vi "povorot_na_vneshku.vi"() -> ()   [LabVIEW 2017]
uses:
  <vilib>/userdefined/High Color/IMAQdx.ctl
  <vilib>/vision/driver/NI_Vision_Acquisition_Software.lvlib
panel:
  out "X":sgl
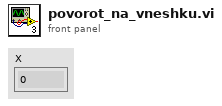
[diagram p1: front panel]
types:
  T1 = typedef "IMAQdx.ctl" = refnum<k21>
  T2 = typedef "IMAQ Image.ctl" = refnum<image>
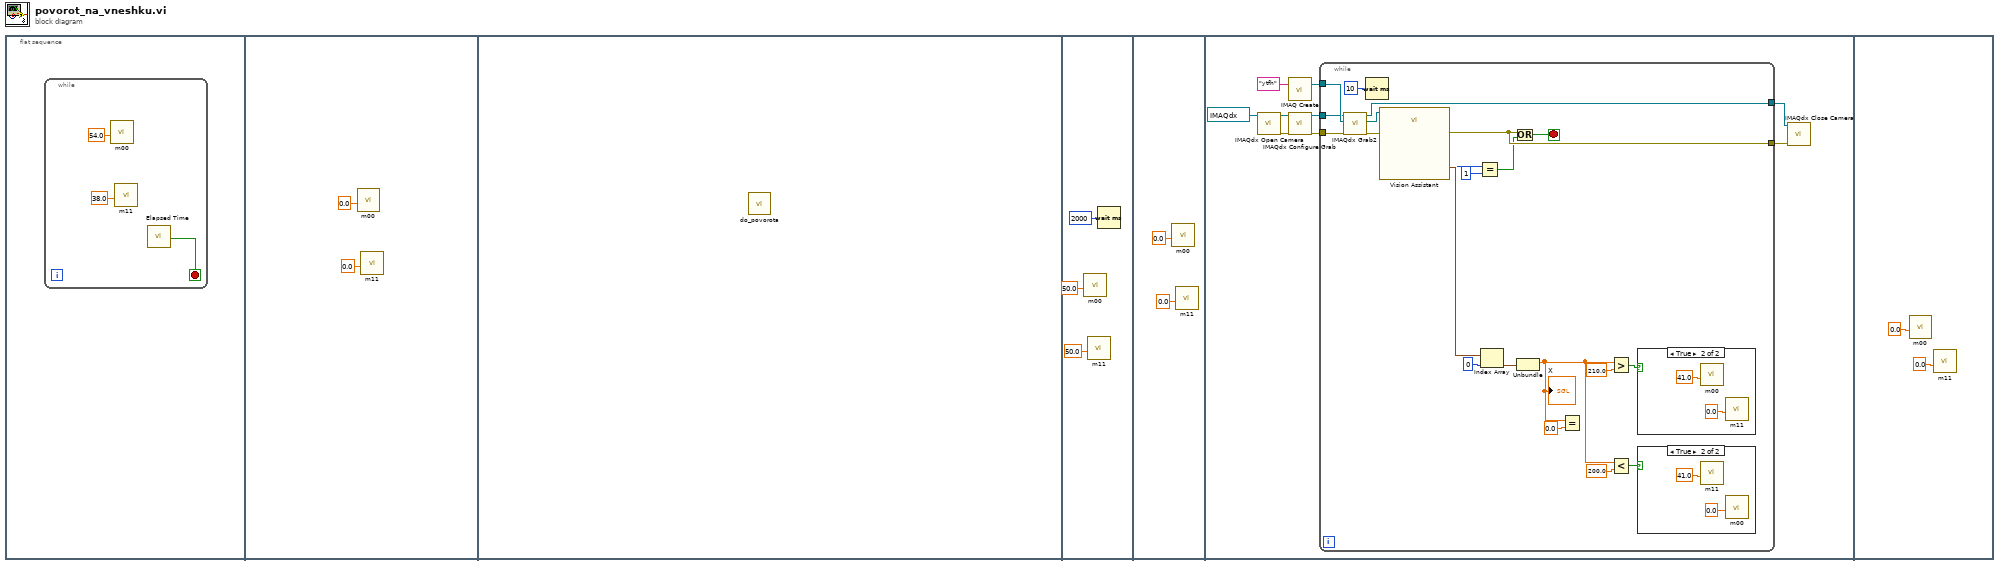
[diagram p0: block diagram]
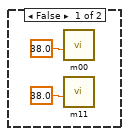
[diagram p2: hidden frame]
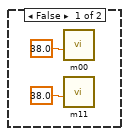
[diagram p3: hidden frame]
diagram:
  n1 = flat-sequence {
    frame #0 {
      n2 = while {
        stop <- w1 stop-if-true
        n3 = call "m00.vi"("position"=54.0) -> ()  [unwired: 10 in, 1 out]
        n4 = call "m11.vi"("position"=38.0) -> ()  [unwired: 10 in, 1 out]
        n5 = call "Elapsed Time"() -> ("Time has Elapsed"=w1:bool)  [unwired: 12 in, 7 out]
      }
    }
    frame #1 {
      n6 = call "m00.vi"("position"=0.0) -> ()  [unwired: 10 in, 1 out]
      n7 = call "m11.vi"("position"=0.0) -> ()  [unwired: 10 in, 1 out]
    }
    frame #2 {
      n8 = call "do_povorota.vi"() -> ()  [unwired: 12 in]
    }
    frame #3 {
      n9 = call "m00.vi"("position"=50.0) -> ()  [unwired: 10 in, 1 out]
      n10 = call "m11.vi"("position"=50.0) -> ()  [unwired: 10 in, 1 out]
      n11 = Wait (ms)(milliseconds to wait=u32 2000) -> ()  [unwired: 1 out]
    }
    frame #4 {
      n12 = call "m00.vi"("position"=0.0) -> ()  [unwired: 10 in, 1 out]
      n13 = call "m11.vi"("position"=0.0) -> ()  [unwired: 10 in, 1 out]
    }
    frame #5 {
      n14 = call <vilib>:"IMAQdx Open Camera.vi"("Session In"=T1 "cam1") -> ("error out"=w16:errorcluster, "Session Out"=w15:T1)  [unwired: 9 in]
      n15 = call "IMAQ Create"("Image Name"="ytfh") -> ("New Image"=w13:T2)  [unwired: 4 in, 1 out]
      n16 = call <vilib>:"IMAQdx Configure Grab.vi"("error in"=w16, "Session In"=w15) -> ("error out"=w17:errorcluster, "Session Out"=w14:T1)  [unwired: 8 in]
      n17 = while {
        tunnel: w17 -> [w35]
        tunnel: w13 -> [w34]
        tunnel: w14 -> [w33]
        tunnel: [w32] -> w19
        tunnel: [w30] -> w18
        stop <- w31 stop-if-true
        n18 = call <vilib>:"IMAQdx Grab2.vi"("error in"=w35, "Image In"=w34, "Session In"=w33) -> ("error out"=w37:errorcluster, "Image Out"=w36:T2, "Session Out"=w32:T1)  [unwired: 5 in, 1 out]
        n19 = Wait (ms)(milliseconds to wait=u32 10) -> ()  [unwired: 1 out]
        n20 = call "Vision Assistant"("Image In"=w36, "error in"=w37) -> ("Edges Coordinates (Edge Detector 1)"=w40:cluster{"X":sgl, "Y":sgl}[], "Number of Matches (Color Location 1)"=w22:i32, "error out"=w30:errorcluster)  [unwired: 22 in, 1 out]
        n21 = Equal?(x=w22, y=1) -> (x = y?=w21:bool)
        n22 = Index Array(array=w40, index=0) -> (element=w39:cluster{"X":sgl, "Y":sgl})
        n23 = Or(x=w30, y=w21) -> (x .or. y?=w31:bool)
        n24 = Unbundle(w39) -> ("X"=w25:sgl)  [unwired: 1 out]
        "X" <- w25
        n25 = Equal?(x=w25, y=sgl 0.0) -> ()  [unwired: 1 out]
        n26 = Greater?(x=w25, y=sgl 210.0) -> (0:w28:bool)
        n27 = Less?(x=w25, y=sgl 200.0) -> (x < y?=w24:bool)
        n28 = case shown="True" w28 {
          frame False {
            n29 = call "m00.vi"("position"=38.0) -> ()  [unwired: 10 in, 1 out]
            n30 = call "m11.vi"("position"=38.0) -> ()  [unwired: 10 in, 1 out]
          }
          frame True {
            n31 = call "m00.vi"("position"=41.0) -> ()  [unwired: 10 in, 1 out]
            n32 = call "m11.vi"("position"=0.0) -> ()  [unwired: 10 in, 1 out]
          }
        }
        n33 = case shown="True" w24 {
          frame False {
            n34 = call "m00.vi"("position"=38.0) -> ()  [unwired: 10 in, 1 out]
            n35 = call "m11.vi"("position"=38.0) -> ()  [unwired: 10 in, 1 out]
          }
          frame True {
            n36 = call "m11.vi"("position"=41.0) -> ()  [unwired: 10 in, 1 out]
            n37 = call "m00.vi"("position"=0.0) -> ()  [unwired: 10 in, 1 out]
          }
        }
      }
      n38 = call <vilib>:"IMAQdx Close Camera.vi"("error in"=w18, "Session In"=w19) -> ()  [unwired: 9 in, 1 out]
    }
    frame #6 {
      n39 = call "m00.vi"("position"=0.0) -> ()  [unwired: 10 in, 1 out]
      n40 = call "m11.vi"("position"=0.0) -> ()  [unwired: 10 in, 1 out]
    }
  }
